vi "FTW-Collection-Lookup-String.vi"(0 "Collection":refnum<class "FTW-Collection.lvclass">, 5 "Key":string, 7 "Default Value":string, 11 "error in":errorcluster) -> (4 "Collection out":refnum<class "FTW-Collection.lvclass">, 6 "Found?":bool, 8 "Value":string, 15 "error out":errorcluster)   [LabVIEW 2012, in "FTW-Collection.lvclass"]
uses:
  FTW-Collection.lvclass
  FTW-Collection.lvclass/FTW-Collection.ctl
panel:
  # "Inputs"
  # "Outputs"
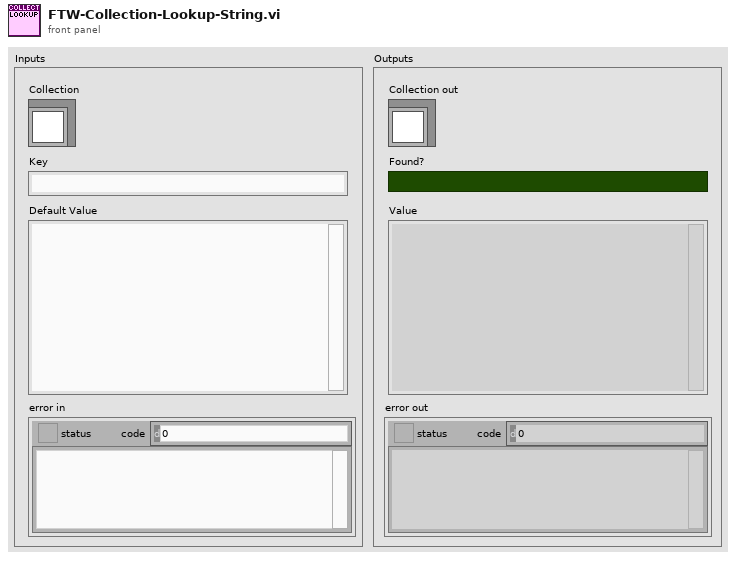
[diagram p1: front panel]
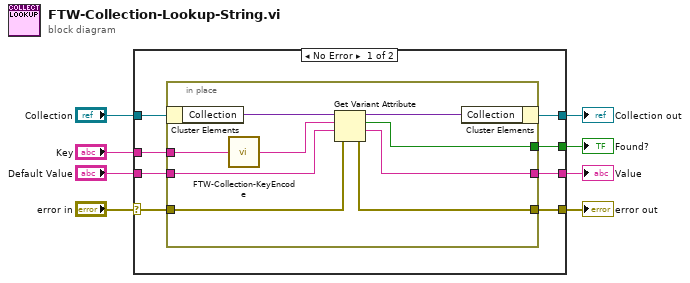
[diagram p0: block diagram]
diagram:
  n1 = case shown="No Error" "error in" {
    selector: "error in" -> [w14 w28]
    tunnel: [w10 w28] -> w8
    tunnel: [w11 _] -> w6
    tunnel: "Collection" -> [w16 w27]
    tunnel: "Key" -> [w13 _]
    tunnel: [w15 w27] -> w3
    tunnel: "Default Value" -> [w12 w26]
    tunnel: [w9 w26] -> w1
    frame No Error {
      n2 = in-place {
        in-place-border: w13 -> [w18]
        in-place-border: w14 -> [w23]
        in-place-border: [w22] -> w10
        in-place-border: [w21] -> w11
        in-place-border: w12 -> [w20]
        in-place-border: [w19] -> w9
        n3 = in-place-cluster #1(w16) -> ("Collection"=w25:variant)
        n4 = call "FTW-Collection-KeyEncode.vi"("Key"=w18) -> ("Encoded Key"=w17:string)
        n5 = Get Variant Attribute(Variant=w25, name=w17, default value (empty Variant)=w20, error in=w23) -> (duplicate Variant=w24:variant, found=w21:bool, value=w19:string, error out=w22:errorcluster)
        n6 = in-place-cluster #1("Collection"=w24) -> (w15:refnum<class "FTW-Collection.lvclass">)
      }
    }
    frame Error {
    }
  }
  "error out" <- w8
  "Found?" <- w6
  "Collection out" <- w3
  "Value" <- w1
